vi "Waveform Circular Buffer.vi"(8 "error in":errorcluster, 10 "buffer duration (s)":dbl=10.0, 11 "waveform in":waveform(dbl)) -> (0 "error out":errorcluster, 3 "waveform out":waveform(dbl))   [LabVIEW 2019, in "Instrument.Lockin.lvlib" / "Instrument.DAQ.lvclass"]
doc: "Circular buffer for the waveform datatype, designed for use with continuous data acquisition. The output is a single waveform with duration <b>buffer duration (s)</b>, in seconds. Input waveforms are appended to the end of the output waveform, and elements older than the buffer duration are discarded.\n\nAll input waveforms must have matching <i>dt</i> values. To eliminate drift in sample times, only the most recent trigger timestamp is considered; the trigger timestamp of the output waveform is computed from the most recently input trigger timestamp, the duration of the buffer, and <i>dt</i>. This may introduce jitter in sample times if the difference between the final timestamp of the previous input and the trigger timestamp of the next input are not exactly equal to <i>dt</i>. In this case, the timestamps of the most recent portion of the buffer will be correct, but earlier timestamps will be scaled. In buffered continuous acquisition, waveforms are consecutive and no jitter is introduced by this method.\n\nThe duration of the buffer may be larger than the requested duration if the duration is not an integer multiple of <i>dt</i>.\n\nOn first call, the input waveform fills end of the buffer; earlier values are set to zero, and the trigger timestamp is backdated. For performance reasons, <b>buffer duration (s)</b> is read only on first call."
uses:
  Instrument.DAQ.lvclass
  <vilib>/Waveform/WDTOps.llb/WDT Number of Waveform Samples DBL.vi
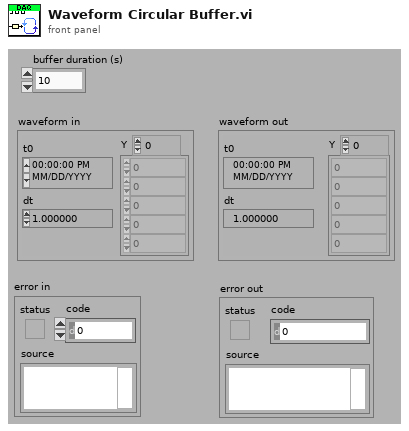
[diagram p1: front panel]
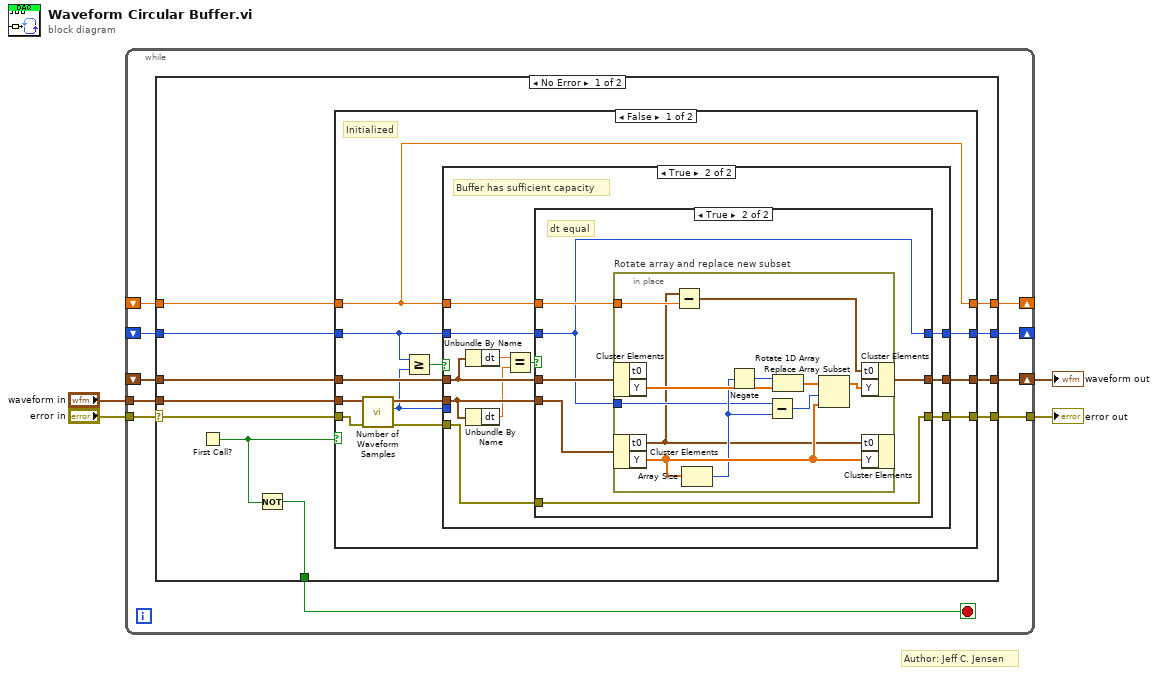
[diagram p0: block diagram]
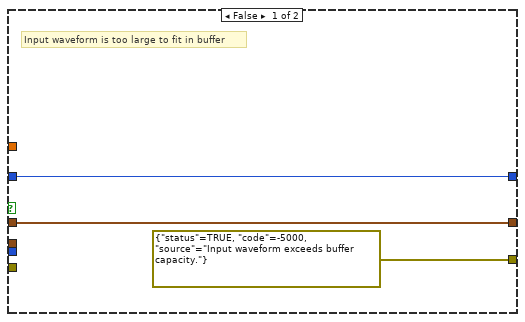
[diagram p2: hidden frame]
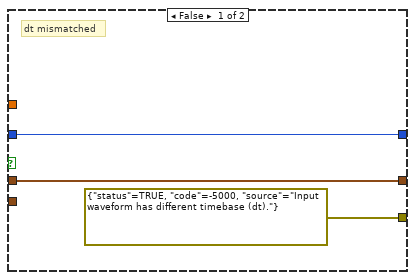
[diagram p3: hidden frame]
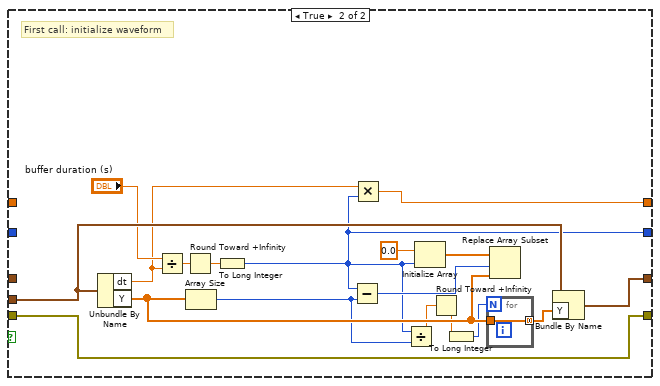
[diagram p4: hidden frame]
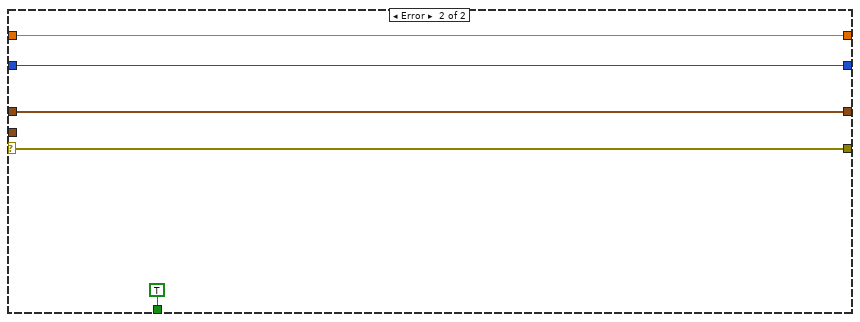
[diagram p5: hidden frame]
diagram:
  # "Author: Jeff C. Jensen"
  n1 = while {
    tunnel: "waveform in" -> [w14]
    tunnel: "error in" -> [w6]
    tunnel: [w12] -> w2
    shift-right: [w13] -> w3
    shift-left: _ -> [w11]
    shift-right: [w10] -> _
    shift-left: _ -> [w9]
    shift-right: [w8] -> _
    shift-left: _ -> [w7]
    stop <- w5 stop-if-true
    n2 = case shown="No Error" w6 {
      selector: w6 -> [w17 w91]
      tunnel: w14 -> [w25 _]
      tunnel: [w24 w94] -> w13
      tunnel: [w15 TRUE ("First Call?: T/F")] -> w5
      tunnel: [w23 w91] -> w12
      tunnel: w11 -> [w22 w94]
      tunnel: [w21 w93] -> w10
      tunnel: w9 -> [w20 w93]
      tunnel: [w19 w92] -> w8
      tunnel: w7 -> [w18 w92]
      frame No Error {
        n3 = First Call?() -> (First Call?: T/F=w16:bool)
        n4 = Not(x=w16) -> (.not. x?=w15:bool)
        n5 = case shown="False" w16 {
          tunnel: w25 -> [w34 w88]
          tunnel: [w37 w87] -> w24
          tunnel: w17 -> [w33 w86]
          tunnel: [w36 w86] -> w23
          tunnel: w22 -> [w35 _]
          tunnel: [w30 w75] -> w21
          tunnel: w20 -> [w26 _]
          tunnel: [w29 w79] -> w19
          tunnel: w18 -> [w29 _]
          frame False {
            # "Initialized"
            n6 = call-poly <vilib>:"Number of Waveform Samples.vi"("error in (no error)"=w33, "waveform in"=w34) -> ("error out"=w32:errorcluster, "number of samples"=w27:i32, "waveform out"=w31:waveform(dbl))  [unwired: 7 in]
            n7 = Greater Or Equal?(x=w26, y=w27) -> (x >= y?=w28:bool)
            n8 = case shown="True" w28 {
              tunnel: [w40 w51] -> w37
              tunnel: [errorcluster {"status"=TRUE, "code"=-5000, "source"="Input waveform exceeds buffer capacity."} ("error out") w43] -> w36
              tunnel: w35 -> [w40 w47]
              tunnel: w32 -> [_ w42]
              tunnel: w31 -> [_ w48]
              tunnel: w27 -> [_ _]
              tunnel: w26 -> [w39 w50]
              tunnel: [w39 w44] -> w30
              tunnel: w29 -> [_ w49]
              frame False {
                # "Input waveform is too large to fit in buffer"
              }
              frame True {
                # "Buffer has sufficient capacity"
                n9 = Unbundle By Name(w47) -> ("dt"=w46:dbl)
                n10 = Unbundle By Name(w48) -> ("dt"=w45:dbl)
                n11 = Equal?(x=w46, y=w45) -> (x = y?=w41:bool)
                n12 = case shown="True" w41 {
                  tunnel: [w53 w60] -> w51
                  tunnel: w47 -> [w53 w59]
                  tunnel: w48 -> [_ w58]
                  tunnel: w50 -> [w54 w56]
                  tunnel: w49 -> [_ w57]
                  tunnel: [w54 w56] -> w44
                  tunnel: [errorcluster {"status"=TRUE, "code"=-5000, "source"="Input waveform has different timebase (dt)."} ("error out") w55] -> w43
                  tunnel: w42 -> [_ w55]
                  frame False {
                    # "dt mismatched"
                  }
                  frame True {
                    # "dt equal"
                    n13 = in-place "Rotate array and replace new subset" {
                      in-place-border: w56 -> [w64]
                      in-place-border: w57 -> [w62]
                      n14 = in-place-cluster #1(w59) -> ("Y"=w68:dbl[])  [unwired: 1 out]
                      n15 = in-place-cluster #2(w58) -> ("t0"=w61:timestamp, "Y"=w66:dbl[])
                      n16 = Subtract(x=w61, y=w62) -> (x-y=w63:timestamp)
                      n17 = Array Size(array=w66) -> (size(s)=w65:i32)
                      n18 = Negate(x=w65) -> (-x=w69:i32)
                      n19 = Subtract(x=w64, y=w65) -> (x-y=w67:i32)
                      n20 = Rotate 1D Array(1:w68, 2:w69) -> (0:w71:dbl[])
                      n21 = Replace Array Subset(array=w71, new element=w66, index=w67) -> (w70:dbl[])
                      n22 = in-place-cluster #1("t0"=w63, "Y"=w70) -> (w60:waveform(dbl))
                      n23 = in-place-cluster #2("t0"=w61, "Y"=w66) -> ()  [unwired: 1 out]
                    }
                  }
                }
              }
            }
          }
          frame True {
            # "First call: initialize waveform"
            n24 = Unbundle By Name(w88) -> ("dt"=w80:dbl, "Y"=w77:dbl[])
            n25 = Divide(x="buffer duration (s)", y=w80) -> (x/y=w82:dbl)
            n26 = Round Toward +Infinity(x=w82) -> (ceil(x): smallest int >= x=w81:dbl)
            n27 = Array Size(array=w77) -> (size(s)=w76:i32)
            n28 = To Long Integer(number=w81) -> (32bit integer=w75:i32)
            n29 = Subtract(x=w75, y=w76) -> (x-y=w85:i32)
            n30 = Multiply(x=w80, y=w75) -> (x*y=w79:dbl)
            n31 = Divide(x=w75, y=w76) -> (x/y=w74:dbl)
            n32 = Initialize Array(0.0, w75) -> (w84:dbl[])
            n33 = Round Toward +Infinity(x=w74) -> (ceil(x): smallest int >= x=w73:dbl)
            n34 = To Long Integer(number=w73) -> (32bit integer=w72:i32)
            n35 = for {
              N: w72 -> [_]
              tunnel: [w90] -> w78 mode=concatenating
              tunnel: w77 -> [w90]
            }
            n36 = Replace Array Subset(array=w84, new element=w77, index=w85) -> ()  [unwired: 1 out]
            n37 = Bundle By Name(cluster=w88, "Y"=w78) -> (w87:waveform(dbl))
          }
        }
      }
      frame Error {
      }
    }
  }
  "waveform out" <- w3
  "error out" <- w2
